vi "Get Array Data Variant.vi"(8 "error in (no error)":errorcluster, 11 "Core Plugins Configuration in":refnum<class "Core Plugins Configuration.lvclass">) -> (0 "error out":errorcluster, 1 "data version":T1, 2 "data":variant, 3 "Core Plugins Configuration out":refnum<class "Core Plugins Configuration.lvclass">)   [LabVIEW 2017, in "DSF Core.lvlib" / "Core Plugins Configuration.lvclass"]
uses:
  Core Plugins Configuration.lvclass
  C:/Git/DSF/Core/Classes/Configuration/Configuration.lvclass
  Typedefs/DSF Version Info.ctl
  Configuration.lvclass
  DSF Core.lvlib
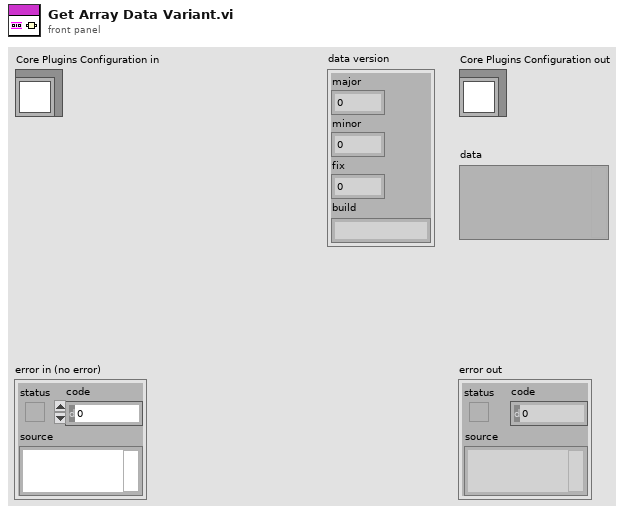
[diagram p1: front panel]
types:
  T1 = typedef "DSF Core.lvlib/DSF Version Info.ctl" = cluster{"major":i32, "minor":i32, "fix":i32, "build":string}
  T2 = typedef "DSF Core.lvlib/Core Plugins Configuration.lvclass/Configuration.ctl" = cluster{"name":string, "components":string[], "cycle timing":T3}
  T3 = typedef "DSF Core.lvlib/DSF Timing Info.ctl" = cluster{"priority":u64, "decimation":u64, "offset":u64}
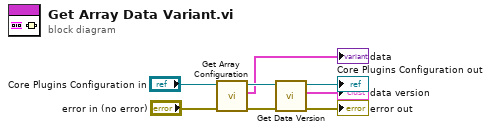
[diagram p0: block diagram]
diagram:
  n1 = call "Get Array Configuration.vi"("error in (no error)"="error in (no error)", "Core Plugins Configuration in"="Core Plugins Configuration in") -> ("error out"=w6:errorcluster, "plugins"=→"data":T2[], "Core Plugins Configuration out"=w5:refnum<class "Core Plugins Configuration.lvclass">)  [unwired: 7 in]
  n2 = call "Get Data Version.vi"("error in (no error)"=w6, "Configuration in"=w5) -> ("error out"=→"error out":errorcluster, "data version"=→"data version":T1, "Configuration out"=→"Core Plugins Configuration out":refnum<class "Core Plugins Configuration.lvclass">)  [unwired: 7 in]
